vi "Update Parameters.vi"(8 "error in (no error)":errorcluster, 10 "Signal Parameters":T1 {"Amplitude" format="%#_2g V"; "Frequency" format="%d Hz"}, 11 "Function Generator Actor in":refnum<class "Function Generator Actor.lvclass">) -> (0 "error out":errorcluster, 3 "Function Generator Actor out":refnum<class "Function Generator Actor.lvclass">)   [LabVIEW 2020, in "Function Generator Actor.lvlib" / "Function Generator Actor.lvclass"]
uses:
  Function Generator Actor.lvclass
  Controls/SignalParamTD.ctl
  Controls/SignalShapeTD.ctl
  Function Generator Actor.lvclass/Function Generator Actor.ctl
  Signal Generation/Signal Generation Messages/ParametersUpdate Msg/ParametersUpdate Msg.lvclass/ParametersUpdate Msg.ctl
  <vilib>/ActorFramework/Message Enqueuer/Message Enqueuer.lvclass/Message Enqueuer.ctl
  <vilib>/ActorFramework/Message Enqueuer/Enqueue.vi
  Signal Generation/Signal Generation Messages/ParametersUpdate Msg/ParametersUpdate Msg.lvclass
  C:/Program Files (x86)/National Instruments/LabVIEW 2020/vi.lib/ActorFramework/Message/Message.lvclass
  <vilib>/ActorFramework/Message Priority Queue/Priority Enqueue.vi
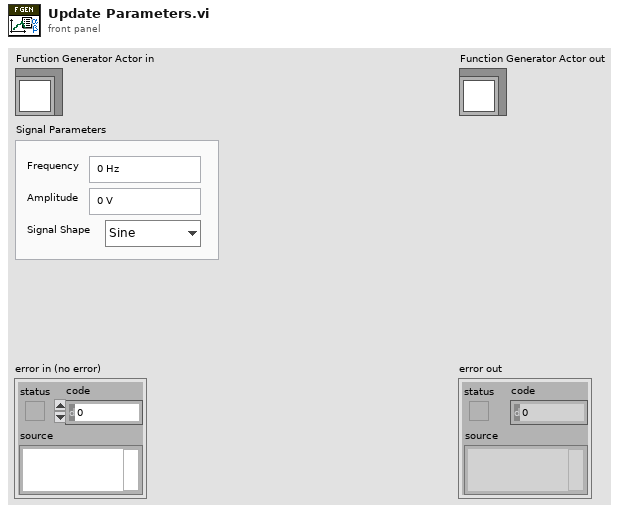
[diagram p1: front panel]
types:
  T1 = typedef "SignalParamTD.ctl" = cluster{"Frequency":u32, "Amplitude":dbl, "Signal Shape":T2}
  T2 = typedef "SignalShapeTD.ctl" = enum16{"Sine", "Square", "Triangle"}
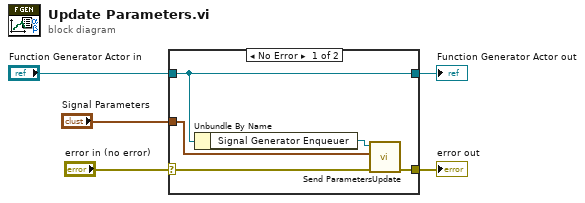
[diagram p0: block diagram]
diagram:
  n1 = case shown="No Error" "error in (no error)" {
    selector: "error in (no error)" -> [w9 w12]
    tunnel: [w8 w12] -> w4
    tunnel: [w10 w11] -> w2
    tunnel: "Function Generator Actor in" -> [w10 w11]
    tunnel: "Signal Parameters" -> [w6 _]
    frame No Error {
      n2 = Unbundle By Name(w10) -> ("Signal Generator Enqueuer"=w7:refnum<class "Message Enqueuer.lvclass">)
      n3 = call "Send ParametersUpdate.vi"("error in (no error)"=w9, "Signal Parameters"=w6, "Message Enqueuer"=w7) -> ("error out"=w8:errorcluster)  [unwired: 7 in, 1 out]
    }
    frame Error {
    }
  }
  "error out" <- w4
  "Function Generator Actor out" <- w2
